vi "Send pcfs_DO_perform_scan.vi"(7 "Message Priority (Normal)":T4=enum."Normal", 8 "error in (no error)":errorcluster, 10 "scan_position_settings":T1={"Center Pos. (mm)"=0.0, "Increment (mm)"=0.0, "Steps"=0.0, "Dither Dist (nm)"=0.0, "Dither Period (s)"=0.0, "Cycles"=0.0, "Record Type"=enum."hdf5", "Save Path"=path "", "Stage Number"=enum."1", "File Notes"="", "Mode"=2, "overwrite"=FALSE, "custom_path"=FALSE, "custom_positions"=[]} {"Mode" items=["T2"=2, "T3"=3]}, 11 "Message Enqueuer":refnum<class "Message Enqueuer.lvclass">) -> (0 "error out":errorcluster, 3 "Message Enqueuer out":refnum<class "Message Enqueuer.lvclass">)   [LabVIEW 2015, in "pcfs_DO_perform_scan Msg.lvclass"]
doc: "This VI sends the message to an actor."
uses:
  pcfs_DO_perform_scan Msg.lvclass
  <vilib>/ActorFramework/Message Enqueuer/Message Enqueuer.lvclass
  <vilib>/ActorFramework/Message Enqueuer/Message Priority.ctl
  PCFS/pcfs_settings.ctl
  Scan/scan_record.ctl
  Detector_Class/Picoquant/Hydraharp/hydraharp_panel/hpanel_acq_modes.ctl
  pcfs_DO_perform_scan Msg.lvclass/pcfs_DO_perform_scan Msg.ctl
  <vilib>/ActorFramework/Message Enqueuer/Message Enqueuer.lvclass/Message Enqueuer.ctl
  <vilib>/ActorFramework/Message Priority Queue/Priority Enqueue.vi
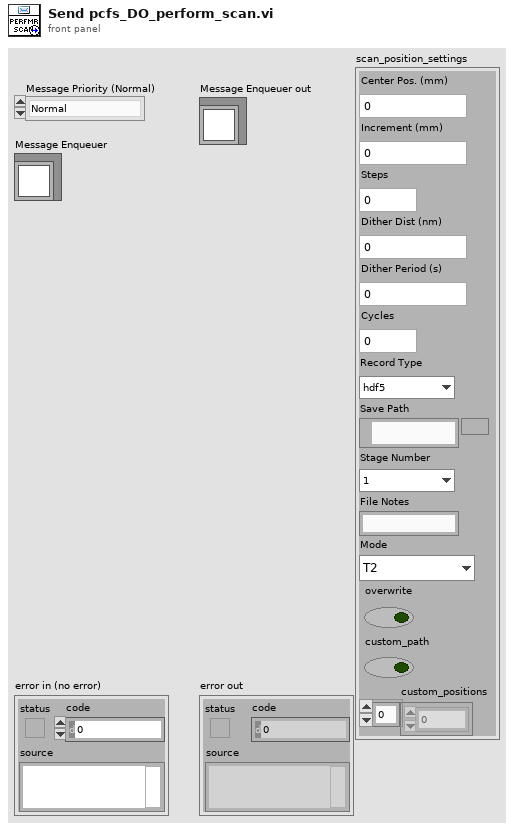
[diagram p1: front panel]
types:
  T1 = typedef "pcfs_settings.ctl" = cluster{"Center Pos. (mm)":dbl, "Increment (mm)":dbl, "Steps":dbl, "Dither Dist (nm)":dbl, "Dither Period (s)":dbl, "Cycles":dbl, "Record Type":T2, "Save Path":path, "Stage Number":enum16{"1", "2"}, "File Notes":string, "Mode":T3, "overwrite":bool, "custom_path":bool, "custom_positions":dbl[]}
  T2 = typedef "scan_record.ctl" = enum16{"hdf5", "legacy", "None"}
  T3 = typedef "hpanel_acq_modes.ctl" = u16
  T4 = typedef "Actor Framework.lvlib/Message Enqueuer.lvclass/Message Priority.ctl" = enum16{"Low", "Normal", "High"}
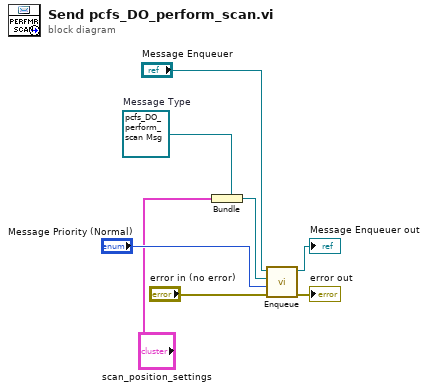
[diagram p0: block diagram]
diagram:
  w5 = refnum<class "pcfs_DO_perform_scan Msg.lvclass"> refnum  # Message Type
  n1 = Bundle(cluster=w5, "scan_position_settings") -> (w4:refnum<class "pcfs_DO_perform_scan Msg.lvclass">)
  n2 = call <vilib>:"Enqueue.vi"("error in (no error)"="error in (no error)", "Message Priority (Normal)"="Message Priority (Normal)", "Message"=w4, "Message Enqueuer in"="Message Enqueuer") -> ("error out"=→"error out":errorcluster, "Message Enqueuer out"=→"Message Enqueuer out":refnum<class "Message Enqueuer.lvclass">)  [unwired: 6 in]
